vi "Launcher.vi"() -> ()   [LabVIEW 2024]
uses:
  Interactor/Interactor.lvclass
  <vilib>/MGI/Panel Manager/Panel/Window Position/Reference Position/Ref VI/Ref VI.lvclass
  <vilib>/MGI/Panel Manager/Panel Actor/Panel Actor/Panel Actor.lvclass
  <vilib>/MGI/Panel Manager/Panel/Panel.lvlib
  <vilib>/MGI/Panel Manager/Panel/Window Position/Reference Position/Horizontal Alignment.ctl
  <vilib>/MGI/Panel Manager/Panel/Window Position/Reference Position/Reference Position.lvclass
  <vilib>/MGI/Panel Manager/Panel/Window Position/Reference Position/Vertical Alignment.ctl
  <vilib>/MGI/Panel Manager/Panel/Window Position/Reference Position/Alignment.ctl
  HAL/Source/Communicator/Communicator.lvclass
  HAL/HAL-Devices/Source/Configure Strategies/PCAN-USB Strategies/PCAN-USB Read-Write Raw CAN Frame Strategy/PCAN Read-Write Raw CAN Frame Strategy.lvclass
  HAL/Source/Config from JSON/Config from JSON.lvclass
  <vilib>/MGI/Panel Manager/Panel Actor/Panel Actor/Launch Root Panel Window.vi
  <vilib>/MGI/Panel Manager/Panel/Window Position/Reference Position/Ref VI/Ref VI.vi
panel:
  out "Error Out":errorcluster
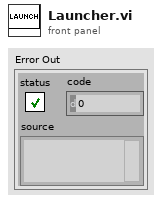
[diagram p1: front panel]
types:
  T1 = typedef "Panel.lvlib/Reference Position.lvclass/Alignment.ctl" = cluster{"Horizontal":T2, "Vertical":T3}
  T2 = typedef "Panel.lvlib/Reference Position.lvclass/Horizontal Alignment.ctl" = enum16{"Left", "Center", "Right"}
  T3 = typedef "Panel.lvlib/Reference Position.lvclass/Vertical Alignment.ctl" = enum16{"Top", "Center", "Bottom"}
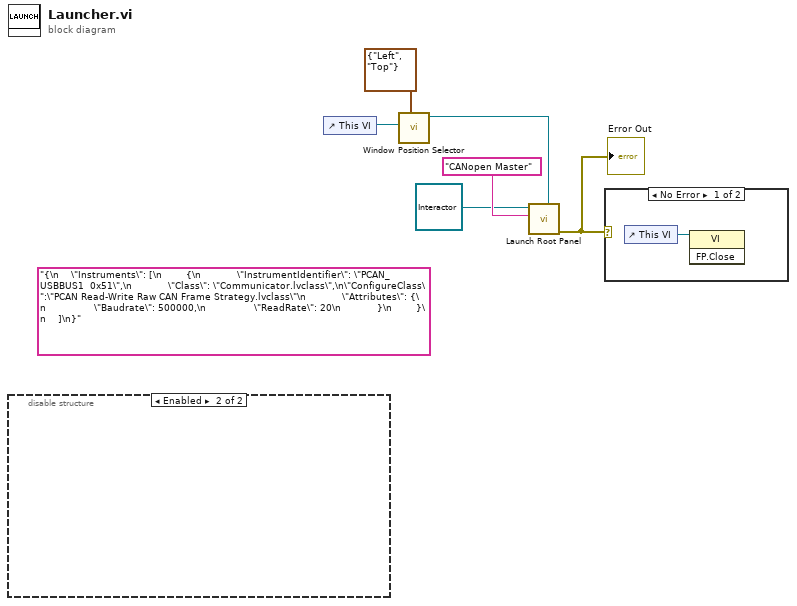
[diagram p0: block diagram]
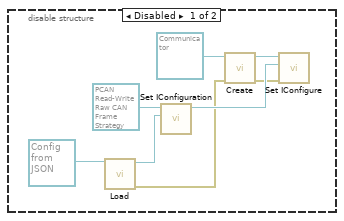
[diagram p2: hidden frame]
diagram:
  (unwired) "{\n    \"Instruments\": [\n        {\n            \"InstrumentIdentifier\": \"PCAN_USBBUS1  0x51\",\n            \"Class\": \"Communicator.lvclass\",\n\"ConfigureClass\":\"PCAN Read-Write Raw CAN Frame Strategy.lvclass\"\n            \"Attributes\": {\n                \"Baudrate\": 500000,\n                \"ReadRate\": 20\n            }\n        }\n    ]\n}" ("<JSON>CFG")
  n1 = disable-structure shown="Enabled" {
    frame Disabled {
      n2 = call-dynamic "Load.vi"("Config From JSON in"=refnum<class "Config from JSON.lvclass"> refnum ("Config from JSON.lvclass")) -> ("error out"=w8:errorcluster, "Config From JSON out"=w11:refnum<class "Config from JSON.lvclass">)  [unwired: 9 in]
      n3 = call-dynamic "Set IConfiguration.vi"("IConfiguration"=w11, "PCAN-USB Read-Write Raw CAN Frame Strategy in"=refnum<class "PCAN Read-Write Raw CAN Frame Strategy.lvclass"> refnum ("PCAN-USB Read-Write Raw CAN Frame Strategy")) -> ("PCAN-USB Read-Write Raw CAN Frame Strategy out"=w13:refnum<class "PCAN Read-Write Raw CAN Frame Strategy.lvclass">)  [unwired: 9 in]
      n4 = call-dynamic "Create.vi"("Error In"=w8, "reference in"=refnum<class "Communicator.lvclass"> refnum ("Communicator")) -> ("Error Out"=w7:errorcluster, "reference out"=w9:refnum<class "Communicator.lvclass">)  [unwired: 8 in]
      n5 = call-dynamic "Set IConfigure.vi"("Error In"=w7, "IConfigure"=w13, "Communicator in"=w9) -> ()  [unwired: 7 in, 2 out]
    }
    frame Enabled {
    }
  }
  n6 = control-ref of="This VI"() -> (w3:refnum<vi>)
  n7 = call-poly <vilib>:"Window Position Selector.vi"("Alignment"=T1 {"Horizontal"=enum."Left", "Vertical"=enum."Top"}, "Ref VI"=w3) -> ("Ref VI out"=w6:refnum<class "Ref VI.lvclass">)  [unwired: 8 in, 1 out]
  n8 = call-poly <vilib>:"Launch Root Panel.vi"("Window Position (Maximize First Call)"=w6, "Title"="CANopen Master", "Panel Actor in"=refnum<class "Interactor.lvclass"> refnum ("Interactor.lvlib:Interactor.lvclass")) -> ("Error Out"=w4:errorcluster)  [unwired: 7 in, 1 out]
  "Error Out" <- w4
  n9 = case shown="No Error" w4 {
    frame No Error {
      n10 = control-ref of="This VI"() -> (w15:refnum<vi>)
      n11 = invoke class="VI" method="FP.Close"(reference=w15) -> ()  [unwired: 2 in, 3 out]
    }
    frame Error {
    }
  }
